vi "Draw Filled Triangle.vi"(6 "Fill Colour":u32(colorbox), 8 "Point 3":T1, 9 "Point 2":T1, 10 "Point 1":T1, 11 "Pixel Data in":u32[][](array[numeric])) -> (3 "Pixel Data out":u32[][](array[numeric]))   [LabVIEW 2020, in "Raster.lvlib"]
uses:
  Raster.lvlib
  Point 2D.ctl
  Utility/Utility.lvlib
panel:
  out "Delta Time [s]":dbl format="%.3p"
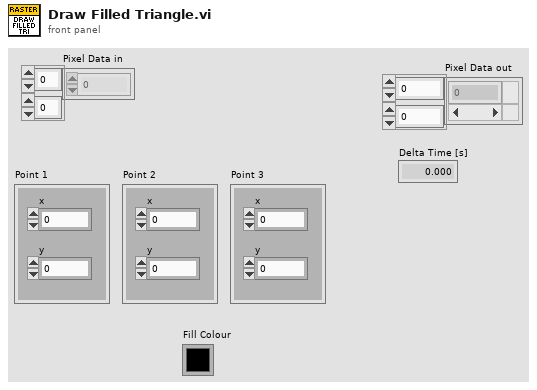
[diagram p1: front panel]
types:
  T1 = typedef "Raster.lvlib/Point 2D.ctl" = cluster{"x":i32, "y":i32}
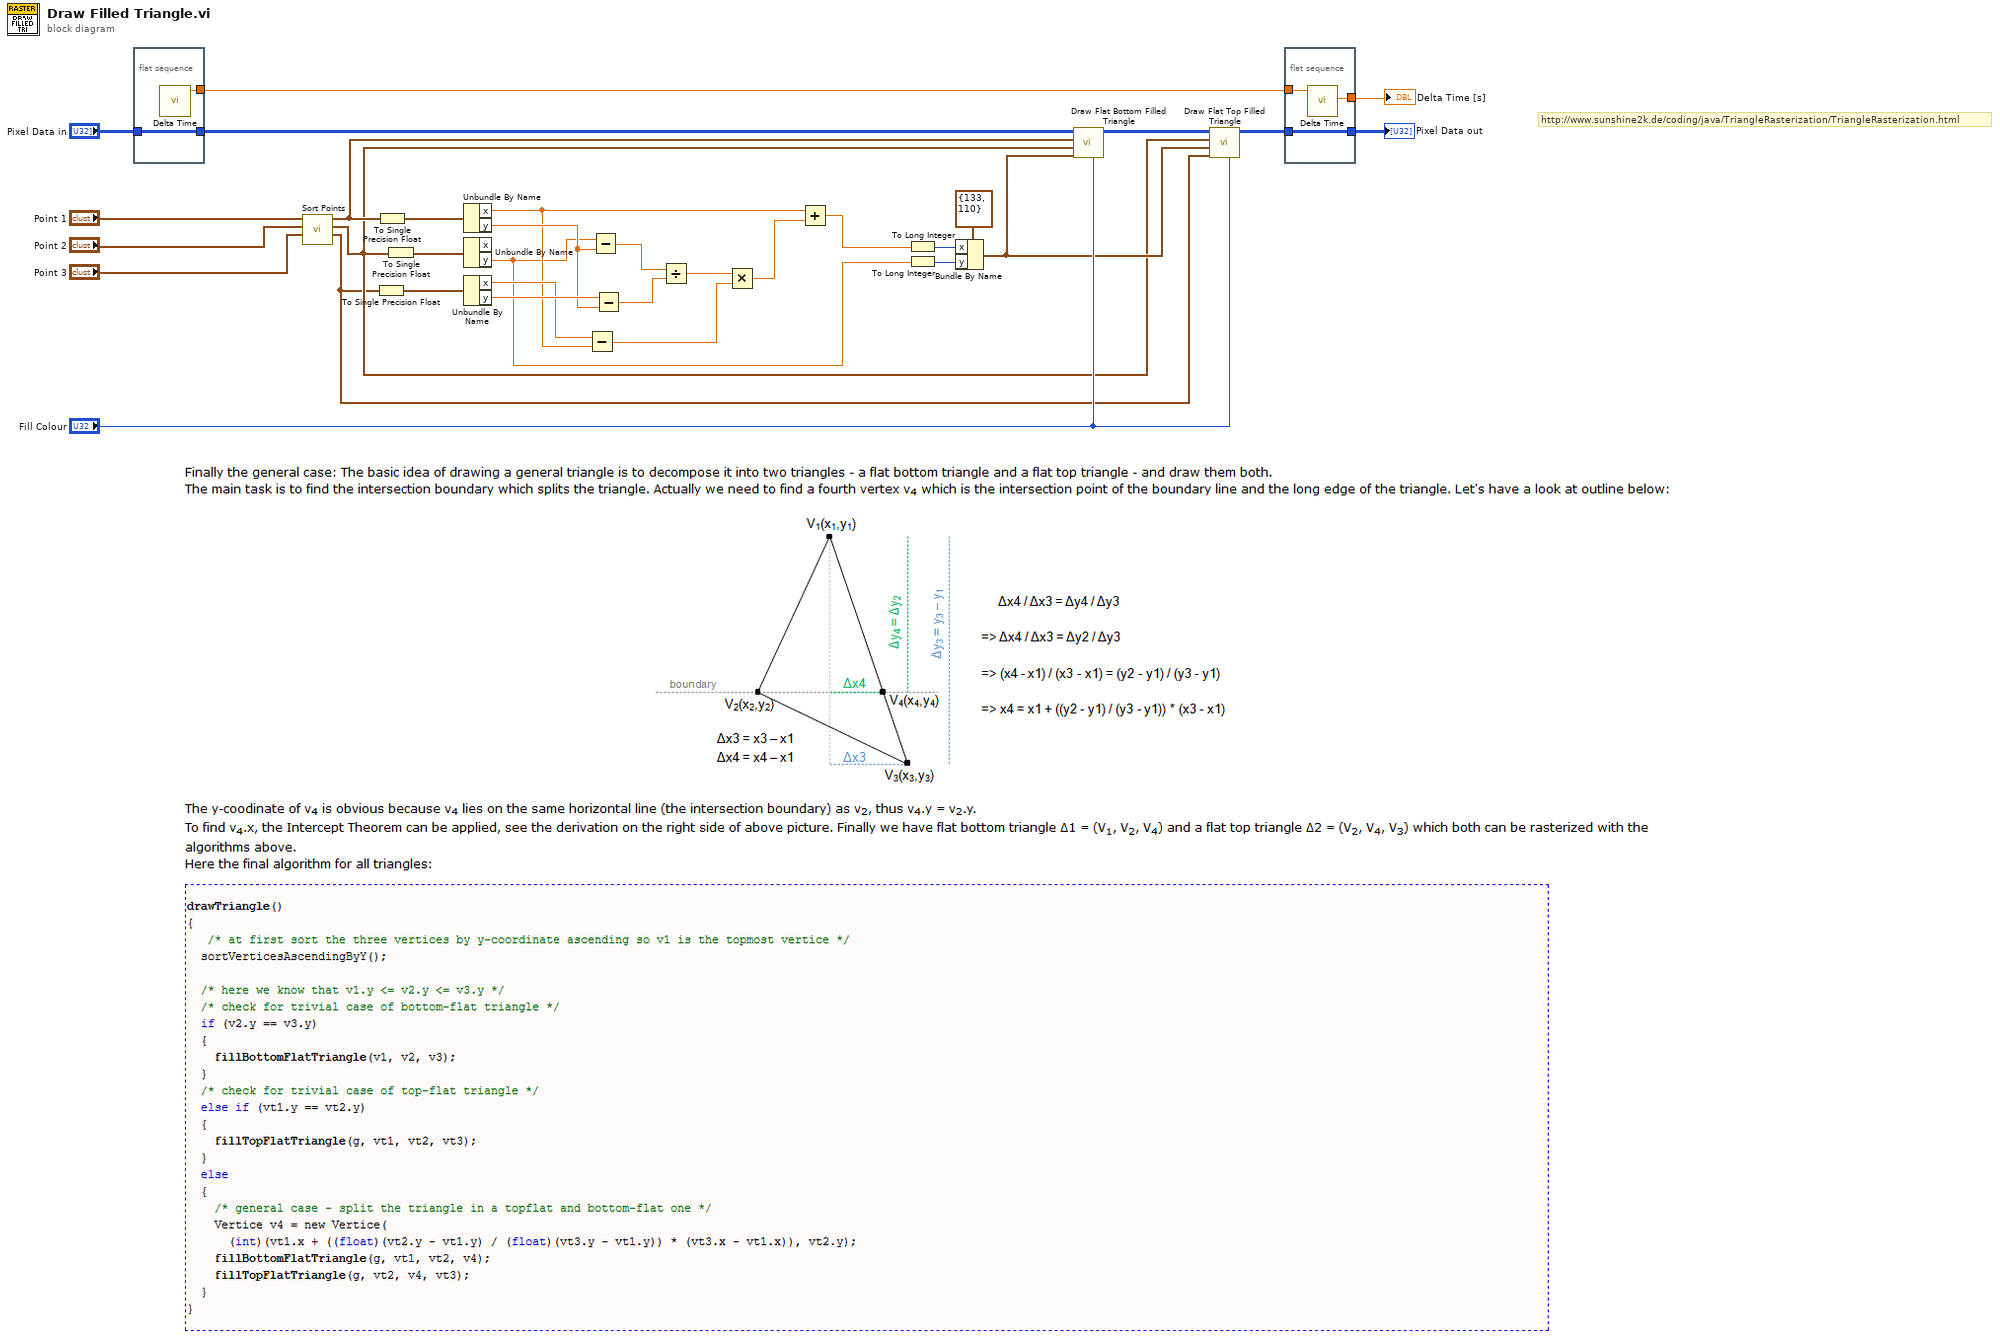
[diagram p0: block diagram]
diagram:
  # "http://www.sunshine2k.de/coding/java/TriangleRasterization/TriangleRasterization.html"
  n1 = flat-sequence {
    tunnel: "Pixel Data in" -> [w34]
    tunnel: [w34] -> w27
    tunnel: [w33] -> w24
    frame #0 {
      n2 = call "Delta Time.vi"() -> ("Relative Seconds Out"=w33:dbl)  [unwired: 10 in, 1 out]
    }
  }
  n3 = call "Sort Points.vi"("Point 3"="Point 3", "Point 2"="Point 2", "Point 1"="Point 1") -> ("Point 3"=w5:T1, "Point 2"=w6:T1, "Point 1"=w7:T1)  [unwired: 6 in]
  n4 = To Single Precision Float(number=w5) -> (single precision float=w18:cluster{"x":sgl, "y":sgl})
  n5 = To Single Precision Float(number=w7) -> (single precision float=w16:cluster{"x":sgl, "y":sgl})
  n6 = To Single Precision Float(number=w6) -> (single precision float=w17:cluster{"x":sgl, "y":sgl})
  n7 = Unbundle By Name(w16) -> ("x"=w14:sgl, "y"=w20:sgl)
  n8 = Unbundle By Name(w17) -> ("y"=w2:sgl)  [unwired: 1 out]
  n9 = Unbundle By Name(w18) -> ("x"=w15:sgl, "y"=w21:sgl)
  n10 = Subtract(x=w15, y=w14) -> (x-y=w11:sgl)
  n11 = Subtract(x=w2, y=w20) -> (x-y=w19:sgl)
  n12 = Subtract(x=w21, y=w20) -> (x-y=w13:sgl)
  n13 = Divide(x=w19, y=w13) -> (x/y=w12:sgl)
  n14 = Multiply(x=w12, y=w11) -> (x*y=w10:sgl)
  n15 = Add(x=w14, y=w10) -> (x+y=w4:sgl)
  n16 = To Long Integer(number=w4) -> (32bit integer=w3:i32)
  n17 = To Long Integer(number=w2) -> (32bit integer=w1:i32)
  n18 = Bundle By Name(cluster=T1 {"x"=133, "y"=110} ("Point 1"), "x"=w3, "y"=w1) -> (w8:T1)
  n19 = call "Draw Flat Bottom Filled Triangle.vi"("Fill Colour"="Fill Colour", "Point 3"=w8, "Point 2"=w6, "Point 1"=w7, "Pixel Data in"=w27) -> ("Pixel Data out"=w22:u32[][])  [unwired: 6 in]
  n20 = call "Draw Flat Top Filled Triangle.vi"("Fill Colour"="Fill Colour", "Point 3"=w5, "Point 2"=w8, "Point 1"=w6, "Pixel Data in"=w22) -> ("Pixel Data out"=w26:u32[][])  [unwired: 6 in]
  n21 = flat-sequence {
    tunnel: w26 -> [w37]
    tunnel: [w37] -> w25
    tunnel: w24 -> [w36]
    tunnel: [w35] -> w23
    frame #0 {
      n22 = call "Delta Time.vi"("Relative Seconds In"=w36) -> ("Delta Time [s]"=w35:dbl)  [unwired: 9 in, 1 out]
    }
  }
  "Pixel Data out" <- w25
  "Delta Time [s]" <- w23
